vi "Test Addition.vi"(11 "Args":string[](array[string])) -> (2 "Output":string, 3 "Exit Code":i32)   [LabVIEW 2021]
uses:
  <vilib>/addons/_JKI Toolkits/Caraya/classes/Test Suite/Define Test Suite (JUnit Report).vi
  <vilib>/addons/_JKI Toolkits/Caraya/classes/Test Suite/Test Suite.lvclass
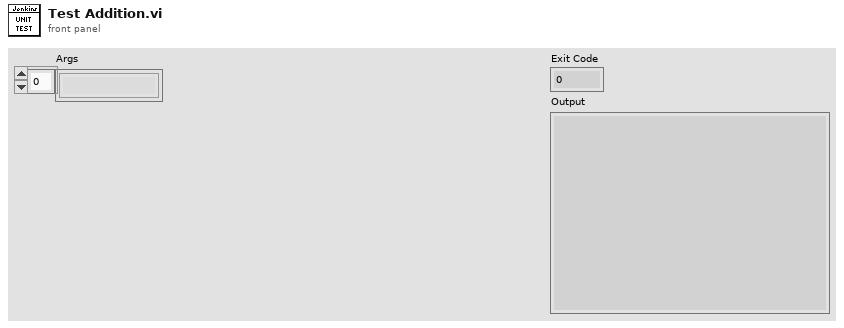
[diagram p1: front panel]
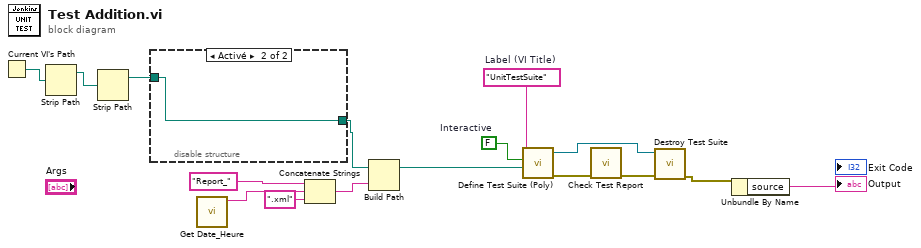
[diagram p0: block diagram]
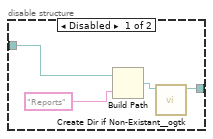
[diagram p2: hidden frame]
diagram:
  w15 = FALSE  # Interactive
  w16 = "UnitTestSuite"  # Label (VI Title)
  n1 = Current VI's Path() -> (path=w7:path)
  n2 = Strip Path(path=w7) -> (stripped path=w6:path)  [unwired: 1 out]
  n3 = Strip Path(path=w6) -> (stripped path=w5:path)  [unwired: 1 out]
  n4 = disable-structure shown="Activé" {
    disable-tunnel: [w18 w21] -> w12
    disable-tunnel: w5 -> [w17 w21]
    frame Disabled {
      n5 = Build Path(base path=w17, name or relative path="Reports") -> (appended path=w19:path)
      n6 = call <userlib>:"Create Dir if Non-Existant__ogtk.vi"("Directory Path"=w19) -> ("dup Directory Path"=w18:path)  [unwired: 8 in, 2 out]
    }
    frame Enabled {
    }
  }
  n7 = call "Get Date_Heure.vi"() -> ("Date_Heure"=w9:string)  [unwired: 11 in]
  n8 = Concatenate Strings("Report_" ("Report Path"), w9, ".xml" ("chaîne")) -> (w11:string)
  n9 = Build Path(base path=w12, name or relative path=w11) -> (appended path=w14:path)
  n10 = call-poly <vilib>:"Define Test Suite (Poly).vi"("Report Path"=w14, "Interactive"=w15, "Label (VI Title)"=w16) -> ("error out"=w4:errorcluster, "Test Suite"=w8:refnum<class "Test Suite.lvclass">)  [unwired: 6 in, 1 out]
  n11 = call "Check Test Report.vi"("error in (no error)"=w4) -> ("error out"=w3:errorcluster)  [unwired: 10 in]
  n12 = call-dynamic "Destroy Test Suite.vi"("error in (no error)"=w3, "Test Suite in"=w8) -> ("error out"=w2:errorcluster)  [unwired: 8 in, 1 out]
  n13 = Unbundle By Name(w2) -> ("source"=→"Output":string)
